vi "p6y3.vi"() -> ()   [LabVIEW 2020]
uses:
  Punkt.ctl
panel:
  out "XY Graph":cluster{"X":dbl, "Y":dbl}[](graph)
  out "appended array":T1[](array[typedef])
  out "data out":string
  in  "Stop":bool
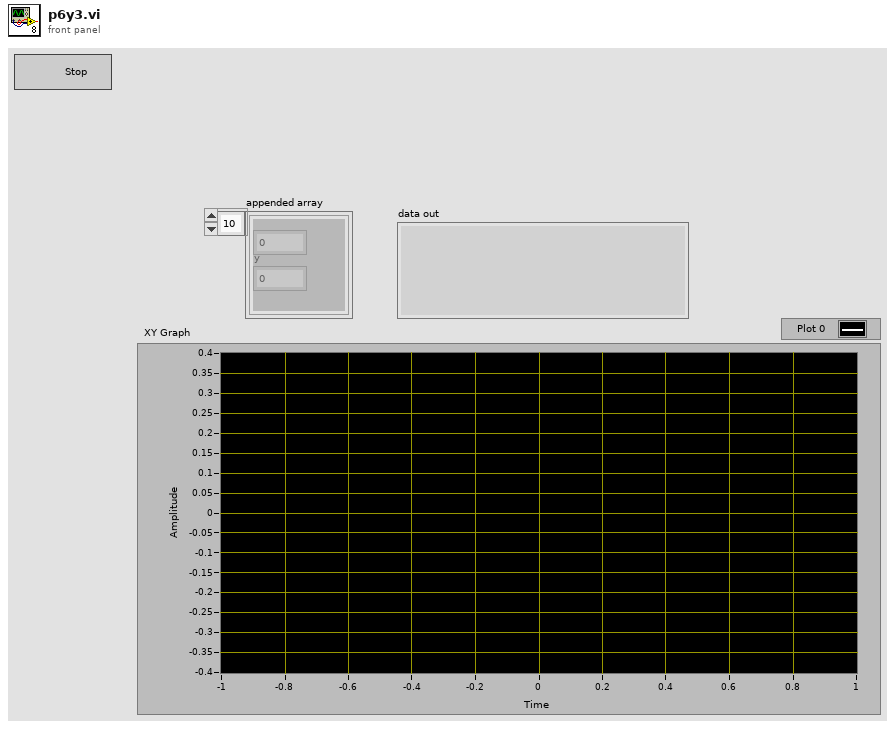
[diagram p1: front panel]
types:
  T1 = typedef "Punkt.ctl" = cluster{"x":dbl, "y":dbl}
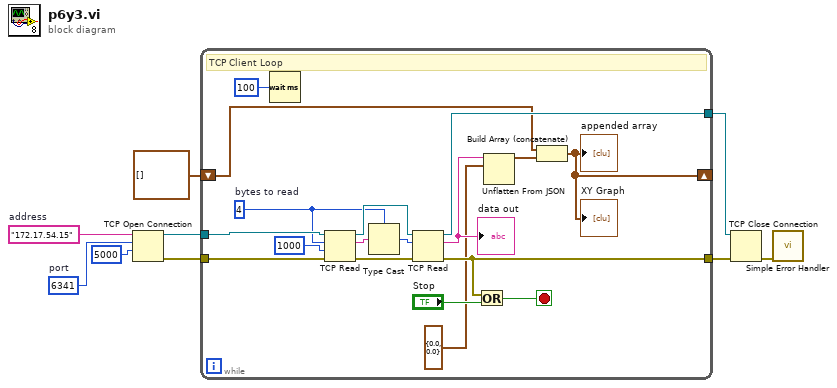
[diagram p0: block diagram]
diagram:
  w6 = u16 6341  # port
  w7 = "172.17.54.15"  # address
  n1 = TCP Open Connection(address=w7, remote port or service name=w6, timeout ms (60000)=5000) -> (connection ID=w9:refnum<k5>, error out=w8:errorcluster)  [unwired: 2 in]
  n2 = while {
    tunnel: w8 -> [w23]
    tunnel: w9 -> [w24]
    tunnel: [w18] -> w5
    tunnel: [w17] -> w4
    shift-right: [w10] -> _
    shift-left: T1[] [] ("Array") -> [w11]
    stop <- w20 stop-if-true
    w22 = 4  # bytes to read
    # "TCP Client Loop"
    n3 = Wait (ms)(milliseconds to wait=u32 100) -> ()  [unwired: 1 out]
    n4 = TCP Read(connection ID=w24, bytes to read=w22, error in (no error)=w23, 9:1000 ("timeout ms (25000)")) -> (connection ID out=w26:refnum<k5>, data out=w27:string, error out=w25:errorcluster)  [unwired: 1 in]
    n5 = Type Cast(type=w22, x=w27) -> (*(type *) &x=w16:i32)
    n6 = TCP Read(connection ID=w26, bytes to read=w16, error in (no error)=w25) -> (connection ID out=w18:refnum<k5>, data out=w14:string, error out=w17:errorcluster)  [unwired: 2 in]
    "data out" <- w14
    n7 = Or(x=w17, y="Stop") -> (x .or. y?=w20:bool)
    n8 = Unflatten From JSON(JSON string=w14, type and defaults=T1 {"x"=0.0, "y"=0.0} ("Cluster")) -> (value=w12:T1)  [unwired: 5 in, 1 out]
    n9 = Build Array (concatenate)(w11, w12) -> (w10:T1[])
    "appended array" <- w10
    "XY Graph" <- w10
  }
  n10 = TCP Close Connection(connection ID=w5, error in (no error)=w4) -> (error out=w3:errorcluster)  [unwired: 1 in, 1 out]
  n11 = call <vilib>:"Simple Error Handler.vi"("error in (no error)"=w3) -> ()  [unwired: 4 in, 5 out]
